vi "Restart Command.vi"(8 "error in":errorcluster, 10 "FTE":u64, 11 "CoreOOB_Rx in":refnum<class "CIFCoreOOB_Rx.lvclass">) -> (0 "error out":errorcluster, 3 "CoreOOB_Rx out":refnum<class "CIFCoreOOB_Rx.lvclass">)   [LabVIEW 2021, in "CIFCoreOOB_Rx.lvclass"]
uses:
  CIFCoreOOB_Rx.lvclass
  D:/dev/CIF-LVCore/src/CIFUtilities/CIFOutOfBand/CIFOutOfBand.lvclass
  Typedef/OOB Core Commands.ctl
  CIFUtilities/CIFOutOfBand/CIFOutOfBand.lvclass/CIFOutOfBand.ctl
  Typedef/Template Payload.ctl
  CIFCoreOOB_Rx.lvclass/CIFCoreOOB_Rx.ctl
  CIFUtilities/CIFOutOfBand/CIFOutOfBand.lvclass
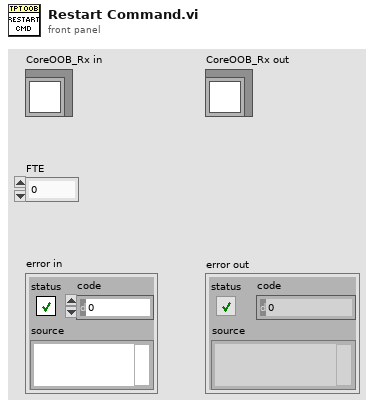
[diagram p1: front panel]
types:
  T1 = typedef "CIFCoreOOB_Rx.lvclass/OOB Core Commands.ctl" = enum8{"Start", "StartFTE", "Pause", "Stop", "Restart", "RestartFTE", "RefreshStats", "UpdateConfig"}
  T2 = typedef "CIFCoreOOB_Rx.lvclass/Template Payload.ctl" = cluster{"Config Data":variant, "FTE":u64}
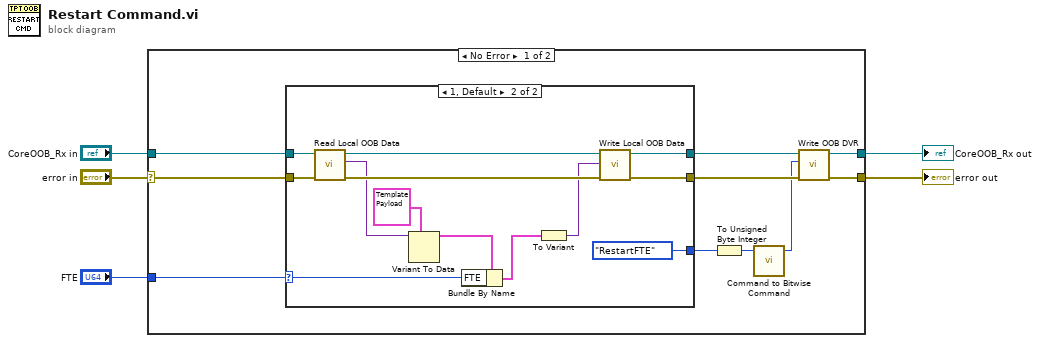
[diagram p0: block diagram]
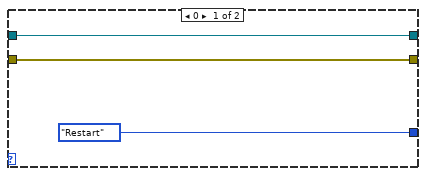
[diagram p2: hidden frame]
diagram:
  n1 = case shown="No Error" "error in" {
    selector: "error in" -> [w12 w33]
    tunnel: [w13 w33] -> w1
    tunnel: "CoreOOB_Rx in" -> [w11 w32]
    tunnel: [w15 w32] -> w2
    tunnel: "FTE" -> [w14 _]
    frame No Error {
      n2 = case shown="1, Default" w14 {
        selector: w14 -> [_ w30]
        tunnel: w11 -> [w18 w28]
        tunnel: [w18 w26] -> w9
        tunnel: [w17 w25] -> w10
        tunnel: w12 -> [w17 w23]
        tunnel: [OOB_Core_Commands."Restart" ("OOB Main Commands") OOB_Core_Commands."RestartFTE" ("OOB Main Commands")] -> w6
        frame 0 {
        }
        frame 1, Default {
          n3 = call "Read Local OOB Data.vi"("error in"=w23, "OOB in"=w28) -> ("error out"=w24:errorcluster, "Local OOB Data"=w21:variant, "OOB in"=w27:refnum<class "CIFCoreOOB_Rx.lvclass">)  [unwired: 7 in]
          n4 = Variant To Data(type=T2 {"Config Data"=variant, "FTE"=0} ("Template Payload"), Variant=w21) -> (data=w31:T2)  [unwired: 1 in, 1 out]
          n5 = Bundle By Name(cluster=w31, "FTE"=w30) -> (w29:T2)
          n6 = To Variant(anything=w29) -> (Variant=w22:variant)
          n7 = call "Write Local OOB Data.vi"("error in"=w24, "Local OOB Data"=w22, "OOB in"=w27) -> ("error out"=w25:errorcluster, "OOB in"=w26:refnum<class "CIFCoreOOB_Rx.lvclass">)  [unwired: 7 in]
        }
      }
      n8 = To Unsigned Byte Integer(number=w6) -> (unsigned 8bit integer=w8:u8)
      n9 = call "Command to Bitwise Command.vi"("OOB Command"=w8) -> ("bit command"=w7:u64)  [unwired: 3 in]
      n10 = call "Write OOB DVR.vi"("error in"=w10, "Commands (bitwise)"=w7, "OOB in"=w9) -> ("error out"=w13:errorcluster, "OOB in"=w15:refnum<class "CIFCoreOOB_Rx.lvclass">)  [unwired: 7 in]
    }
    frame Error {
    }
  }
  "error out" <- w1
  "CoreOOB_Rx out" <- w2
